vi "ligits.vi"   [LabVIEW 2011]
uses:
  lights_led_mode.ctl
  roller/roller_globals.vi
  <vilib>/Rock Robotics/WPI/DriverStation/WPI_DriverStationCommDataCacheOp.ctl
types:
  T1 = typedef "WPI_RelayDevRef.ctl" = cluster{"DevStatus":errorcluster, "Relay Channel":T2, "Digital Module":T3, "Relay Direction":T4}
  T2 = typedef "FPGA_DIORelayChannel.ctl" = enum8{"Relay 1", "Relay 2", "Relay 3", "Relay 4", "Relay 5", "Relay 6", "Relay 7", "Relay 8", "Invalid"}
  T3 = typedef "FPGA_TypedefDigitalModule.ctl" = enum16{"Digital Module 1", "Digital Module 2"}
  T4 = typedef "WPI_RelayDirection.ctl" = enum16{"Both directions", "Forward only", "Reverse only"}
  T5 = cluster{"RelayDevRef":T1, "RelayDevRef":T1, "RelayDevRef":T1, "RelayDevRef":T1}
  T6 = typedef "lights_led_mode.ctl" = enum16{"shoot", "balance", "indicator"}
  T7 = typedef "WPI_DriverStationCommDataCacheOp.ctl" = enum16{"Get", "Set", "Init"}
  T8 = cluster{"r_sw_b1":bool, "r_sw_b2":bool, "r_sw_b3":bool, "r_sw_gun":bool, "r_sw_low":bool}
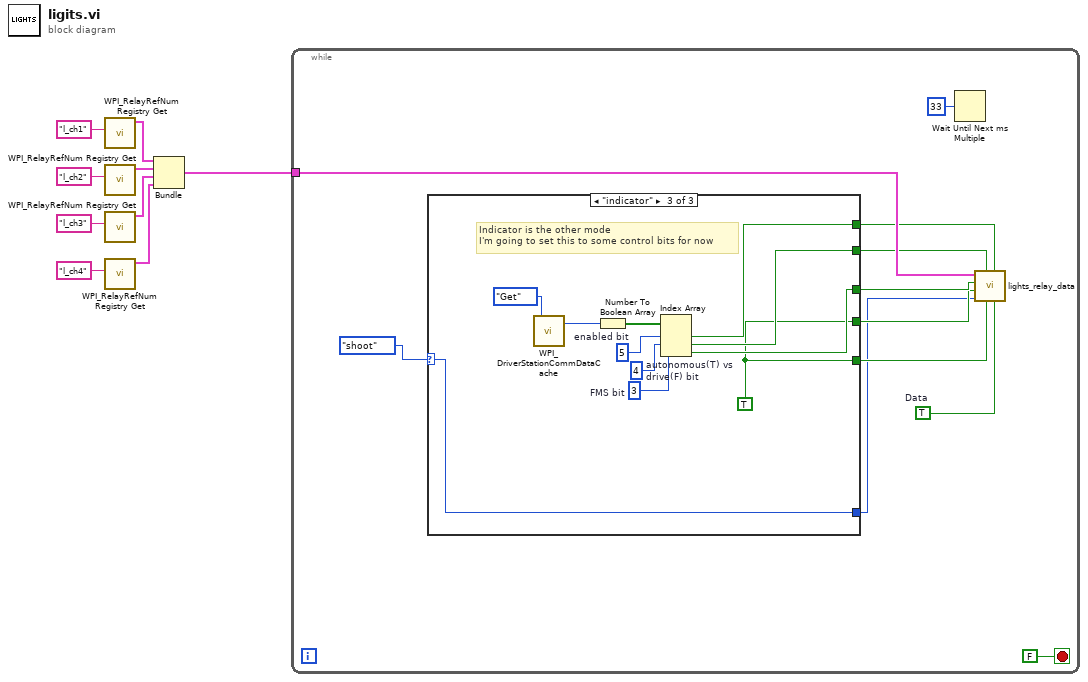
[diagram p0: block diagram]
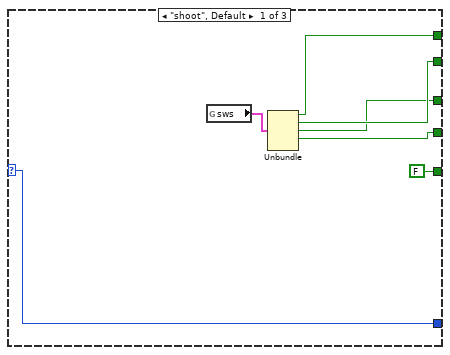
[diagram p2: hidden frame]
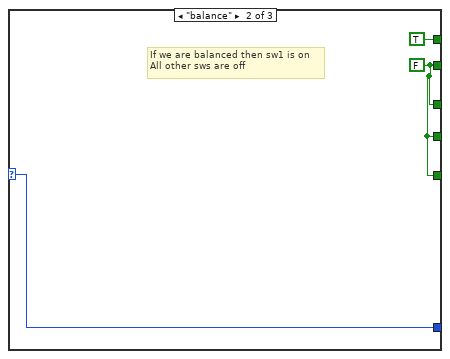
[diagram p3: hidden frame]
diagram:
  n1 = call <vilib>:"WPI_RelayRefNum Registry Get.vi"("refnum name"="l_ch1") -> ("RelayDevRef"=w5:T1)  [unwired: 9 in, 1 out]
  n2 = call <vilib>:"WPI_RelayRefNum Registry Get.vi"("refnum name"="l_ch2") -> ("RelayDevRef"=w4:T1)  [unwired: 9 in, 1 out]
  n3 = call <vilib>:"WPI_RelayRefNum Registry Get.vi"("refnum name"="l_ch3") -> ("RelayDevRef"=w3:T1)  [unwired: 9 in, 1 out]
  n4 = call <vilib>:"WPI_RelayRefNum Registry Get.vi"("refnum name"="l_ch4") -> ("RelayDevRef"=w2:T1)  [unwired: 9 in, 1 out]
  n5 = Bundle("RelayDevRef"=w5, "RelayDevRef"=w4, "RelayDevRef"=w3, "RelayDevRef"=w2) -> (w1:T5)  [unwired: 1 in]
  n6 = while {
    tunnel: w1 -> [w18]
    stop <- FALSE stop-if-true
    w10 = TRUE  # Data
    n7 = case shown="\"indicator\"" lights_led_mode."shoot" ("mode") {
      selector: lights_led_mode."shoot" ("mode") -> [w27 w28 w32]
      tunnel: [w25 TRUE ("r_sw_b1") w36] -> w16
      tunnel: [w24 w30 w35] -> w15
      tunnel: [w23 w30 w33] -> w14
      tunnel: [w22 w30 w31] -> w13
      tunnel: [FALSE ("r_sw_low") w30 w31] -> w12
      tunnel: [w27 w28 w32] -> w11
      frame "shoot", Default {
        n8 = global read "roller_globals.vi" "sws"() -> (w26:T8)
        n9 = Unbundle(w26) -> ("r_sw_b1"=w25:bool, "r_sw_b2"=w24:bool, "r_sw_b3"=w23:bool, "r_sw_gun"=w22:bool)  [unwired: 1 out]
      }
      frame "balance" {
        w30 = FALSE ("r_sw_b2")
        # "If we are balanced then sw1 is on\nAll other sws are off"
      }
      frame "indicator" {
        w31 = TRUE ("r_sw_b2")
        w34 = 3  # FMS bit
        w37 = 4  # autonomous(T) vs drive(F) bit
        w38 = 5  # enabled bit
        # "Indicator is the other mode\nI'm going to set this to some control bits for now"
        n10 = call <vilib>:"WPI_DriverStationCommDataCache.vi"("CommDataCacheOp"=WPI_DriverStationCommDataCacheOp."Get") -> ("ControlBit out"=w40:u8)  [unwired: 18 out]
        n11 = Number To Boolean Array(number=w40) -> (Boolean array=w39:bool[])
        n12 = Index Array(array=w39, index #1=w38, index #2=w37, index #3=w34) -> (element #1=w36:bool, element #2=w35:bool, element #3=w33:bool)
      }
    }
    n13 = Wait Until Next ms Multiple(millisecond multiple=u32 33) -> ()  [unwired: 1 out]
    n14 = call "lights_relay_data.vi"("C2"=w10, "A1"=w16, "C1"=w12, "A2"=w15, "mode"=w11, "B2"=w13, "B1"=w14, "relays"=w18) -> ()  [unwired: 4 in]
  }
